vi "sub_agv_circlepoint_creation.vi"(10 "position":cluster{dbl, dbl}, 11 "lookahed cfg":T1) -> (3 "incircle waypoints":cluster{dbl, dbl}[](array[cluster]))   [LabVIEW 2019]
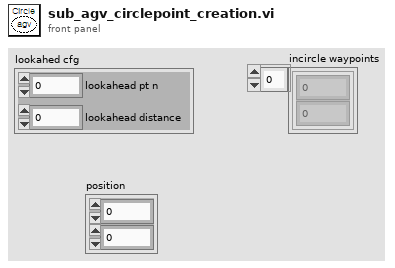
[diagram p1: front panel]
types:
  T1 = cluster{"lookahead pt n":dbl, "lookahead distance":dbl}
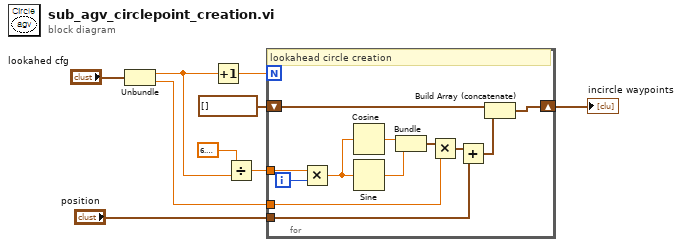
[diagram p0: block diagram]
diagram:
  n1 = Unbundle("lookahed cfg") -> ("lookahead pt n"=w5:dbl, "lookahead distance"=w7:dbl)
  n2 = Increment(x=w5) -> (x+1=w1:dbl)
  n3 = Divide(x=6.283185307179586, y=w5) -> (x/y=w4:dbl)
  n4 = for {
    N: w1 -> [_]
    shift-right: [w18] -> w9
    shift-left: cluster{dbl, dbl}[] [] -> [w17]
    tunnel: w4 -> [w20]
    tunnel: "position" -> [w12]
    tunnel: w7 -> [w10]
    i -> [w21]
    # "lookahead circle creation"
    n5 = Multiply(x=w20, y=w21) -> (x*y=w19:dbl)
    n6 = Cosine(x=w19) -> (cos(x)=w14:dbl)
    n7 = Sine(x=w19) -> (sin(x)=w13:dbl)
    n8 = Bundle(w14, w13) -> (w16:cluster{dbl, dbl})  [unwired: 1 in]
    n9 = Multiply(x=w16, y=w10) -> (x*y=w15:cluster{dbl, dbl})
    n10 = Add(x=w15, y=w12) -> (x+y=w11:cluster{dbl, dbl})
    n11 = Build Array (concatenate)(w17, w11) -> (w18:cluster{dbl, dbl}[])
  }
  "incircle waypoints" <- w9
